vi "Control Init.vi"(7 "VolatusAPI":refnum<class "VolatusAPI.lvclass">, 8 "error in (no error)":errorcluster, 10 "JSON":string, 11 "2WayValve in":refnum<class "2WayValveV.lvclass">) -> (0 "error out":errorcluster, 3 "2WayValve out":refnum<class "2WayValveV.lvclass">)   [LabVIEW 2020, in "VolatusGUIElements.lvlib" / "2WayValveV.lvclass"]
uses:
  2WayValveV.lvclass
  Volatus/VolatusAPI/VolatusAPI.lvclass
  JSON.ctl
  Group Channel.ctl
  Unused Element.ctl
  Values.ctl
  Channel State.ctl
  lv-vecto/Vecto/Group/Group.lvclass
  C:/dev/lv20CE/relink/lv-vecto/Vecto/GroupAbstract/GroupAbstract.lvclass
  2WayValveV.lvclass/2WayValveV.ctl
  5ca493e1-1c63-4061-b4b4-46184d61fbe0.vi
  <vilib>/JDP Science/JSONtext/JSON text to Variant.vi
  <vilib>/JDP Science/JSONtext/LVClass Serializer/JSONtext LVClass Serializer.lvclass
  lv-vecto/Vecto/Channel/Channel.lvclass
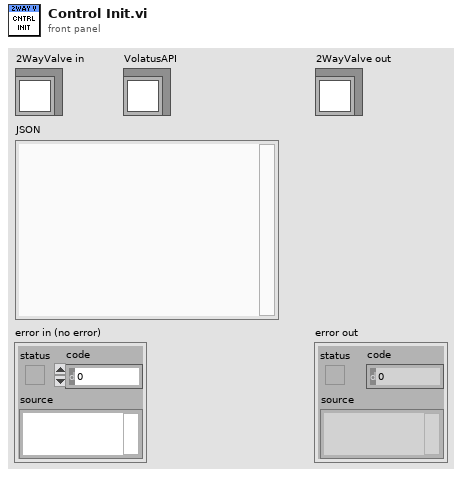
[diagram p1: front panel]
types:
  T1 = typedef "VolatusGUIElements.lvlib/2WayValveV.lvclass/Values.ctl" = cluster{"Command":T2, "CmdFB":T2, "Closed":T2, "Open":T2, "Energized":T2}
  T2 = typedef "VolatusGUIElements.lvlib/2WayValveV.lvclass/Channel State.ctl" = cluster{"Value":bool, "Stale":bool, "Config":bool, "Error":bool, "Prev":bool}
  T3 = typedef "VolatusGUIElements.lvlib/2WayValveV.lvclass/Unused Element.ctl" = cluster{"Command":bool, "Feedback":bool, "Energized":bool}
  T4 = typedef "VolatusGUIElements.lvlib/2WayValveV.lvclass/JSON.ctl" = cluster{"Output":T5, "ClosedFB":T5, "OpenFB":T5, "Energized":T5, "Node":string, "Task":string, "Staleness":dbl}
  T5 = typedef "VolatusGUIElements.lvlib/2WayValveV.lvclass/Group Channel.ctl" = cluster{"Group":string, "Channel":string}
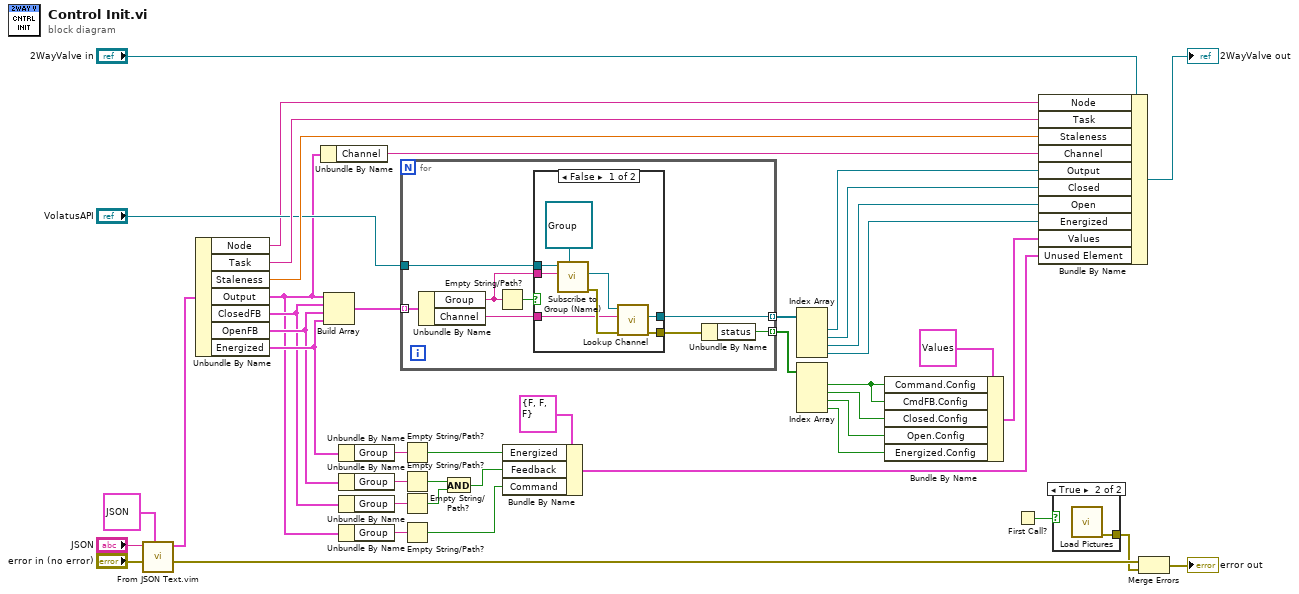
[diagram p0: block diagram]
diagram:
  n1 = call "From JSON Text.vim"("Data Type and Default Value"=T4 {"Output"={"Group"="", "Channel"=""}, "ClosedFB"={"Group"="", "Channel"=""}, "OpenFB"={"Group"="", "Channel"=""}, "Energized"={"Group"="", "Channel"=""}, "Node"="", "Task"="", "Staleness"=0.0} ("JSON"), "error in (no error)"="error in (no error)", "JSON"="JSON") -> ("error out"=w40:errorcluster, "Data out"=w39:T4)  [unwired: 7 in]
  n2 = Unbundle By Name(w39) -> ("Node"=w3:string, "Task"=w17:string, "Staleness"=w8:dbl, "Output"=w2:T5, "ClosedFB"=w36:T5, "OpenFB"=w37:T5, "Energized"=w38:T5)
  n3 = Unbundle By Name(w2) -> ("Channel"=w1:string)
  n4 = Build Array(w2, w36, w37, w38) -> (w25:T5[])
  n5 = Unbundle By Name(w38) -> ("Group"=w35:string)
  n6 = Unbundle By Name(w37) -> ("Group"=w34:string)
  n7 = Unbundle By Name(w36) -> ("Group"=w33:string)
  n8 = Unbundle By Name(w2) -> ("Group"=w32:string)
  n9 = for {
    tunnel: w25 -> [w50] mode=indexing
    tunnel: [w48] -> w24 mode=indexing
    tunnel: [w46] -> w23 mode=indexing
    tunnel: "VolatusAPI" -> [w51]
    n10 = Unbundle By Name(w50) -> ("Group"=w45:string, "Channel"=w49:string)
    n11 = Empty String/Path?(string/path=w45) -> (empty?=w44:bool)
    n12 = case shown="False" w44 {
      tunnel: w51 -> [w58 _]
      tunnel: w45 -> [w56 _]
      tunnel: w49 -> [w54 _]
      tunnel: [w53 _] -> w48
      tunnel: [w52 _] -> w47
      frame False {
        n13 = call "Subscribe to Group (Name).vi"("Group Type"=refnum<class "Group.lvclass"> refnum ("Vecto.lvlib:Group.lvclass"), "Group Name"=w56, "VolatusAPI in"=w58) -> ("error out"=w59:errorcluster, "Group"=w55:refnum<class "Group.lvclass">)  [unwired: 6 in, 1 out]
        n14 = call "Lookup Channel.vi"("error in (no error)"=w59, "Channel Name"=w54, "Group in"=w55) -> ("error out"=w52:errorcluster, "Channel"=w53:refnum<class "Channel.lvclass">)  [unwired: 6 in, 1 out]
      }
      frame True {
      }
    }
    n15 = Unbundle By Name(w47) -> ("status"=w46:bool)
  }
  n16 = Empty String/Path?(string/path=w35) -> (empty?=w30:bool)
  n17 = Empty String/Path?(string/path=w34) -> (empty?=w29:bool)
  n18 = Empty String/Path?(string/path=w33) -> (empty?=w28:bool)
  n19 = Empty String/Path?(string/path=w32) -> (empty?=w26:bool)
  n20 = And(x=w29, y=w28) -> (x .and. y?=w27:bool)
  n21 = Bundle By Name(cluster=T3 {"Command"=FALSE, "Feedback"=FALSE, "Energized"=FALSE} ("Unused Element"), "Energized"=w30, "Feedback"=w27, "Command"=w26) -> (w11:T3)
  n22 = Index Array(array=w24) -> (element #1=w16:refnum<class "Channel.lvclass">, element #2=w15:refnum<class "Channel.lvclass">, element #3=w14:refnum<class "Channel.lvclass">, element #4=w13:refnum<class "Channel.lvclass">)  [unwired: 4 in]
  n23 = Index Array(array=w23) -> (element #1=w21:bool, element #2=w20:bool, element #3=w19:bool, element #4=w18:bool)  [unwired: 4 in]
  n24 = Bundle By Name(cluster=T1 {"Command"={"Value"=FALSE, "Stale"=FALSE, "Config"=FALSE, "Error"=FALSE, "Prev"=FALSE}, "CmdFB"={"Value"=FALSE, "Stale"=FALSE, "Config"=FALSE, "Error"=FALSE, "Prev"=FALSE}, "Closed"={"Value"=FALSE, "Stale"=FALSE, "Config"=FALSE, "Error"=FALSE, "Prev"=FALSE}, "Open"={"Value"=FALSE, "Stale"=FALSE, "Config"=FALSE, "Error"=FALSE, "Prev"=FALSE}, "Energized"={"Value"=FALSE, "Stale"=FALSE, "Config"=FALSE, "Error"=FALSE, "Prev"=FALSE}} ("Values"), "Command.Config"=w21, "CmdFB.Config"=w21, "Closed.Config"=w20, "Open.Config"=w19, "Energized.Config"=w18) -> (w12:T1)
  n25 = First Call?() -> (First Call?: T/F=w7:bool)
  n26 = Bundle By Name(cluster="2WayValve in", "Node"=w3, "Task"=w17, "Staleness"=w8, "Channel"=w1, "Output"=w16, "Closed"=w15, "Open"=w14, "Energized"=w13, "Values"=w12, "Unused Element"=w11) -> (→"2WayValve out":refnum<class "2WayValveV.lvclass">)
  n27 = case shown="True" w7 {
    tunnel: [_ w60] -> w5
    frame False {
    }
    frame True {
      n28 = call "Load Pictures.vi"() -> ("error out"=w60:errorcluster)  [unwired: 11 in]
    }
  }
  n29 = Merge Errors(w40, w5) -> (→"error out":errorcluster)
